vi "Pre Launch Init.vi"(11 "IMediator In":refnum<class "IMediator.lvclass">) -> (0 "error out":errorcluster, 3 "IMediator Out":refnum<class "IMediator.lvclass">)   [LabVIEW 2019, in "IMediator.lvlib" / "IMediator.lvclass"]
doc: "(<B>Filename</B>: Actor Framework.lvlib:Actor.lvclass:Pre Launch Init.vi)\n\nDefines behavior that occurs after the Launch Nested Actor method is invoked but before the actor's Actor Core method begins running.\n\nBy default, this method does nothing. A descendant class may override it to define behavior."
uses:
  <vilib>/gpm_packages/@cs/mva-core/Source/IMediator/IMediator/IMediator.lvclass
  <vilib>/ActorFramework/Actor/Actor.lvclass
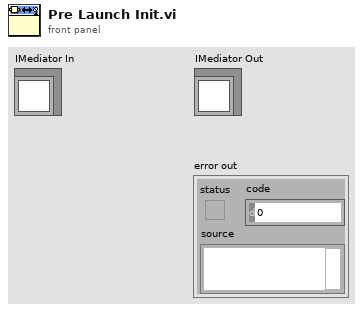
[diagram p1: front panel]
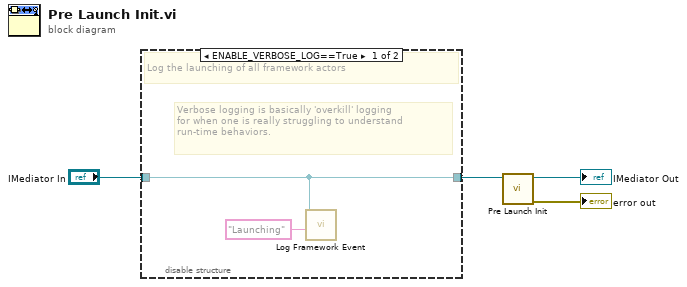
[diagram p0: block diagram]
diagram:
  n1 = disable-structure shown="ENABLE_VERBOSE_LOG==True" {
    disable-tunnel: "IMediator In" -> [w6 w7]
    disable-tunnel: [w6 w7] -> w2
    frame condition #0 {
      # "Verbose logging is basically 'overkill' logging\nfor when one is really struggling to understand\nrun-time behaviors."
      # "Log the launching of all framework actors"
      n2 = call <vilib>:"Log Framework Event.vi"("Data To Log"="Launching", "IMediator In"=w6) -> ()  [unwired: 9 in, 1 out]
    }
    frame condition #1 (active) {
      # "Remove all logging from this method at compile time"
    }
  }
  n3 = call-parent "Pre Launch Init.vi"("Actor in"=w2) -> ("error out"=→"error out":errorcluster, "Actor out"=→"IMediator Out":refnum<class "IMediator.lvclass">)  [unwired: 9 in]
